vi "Main Page.vi"(8 "error in (no error)":errorcluster, 11 "Node Ptr":T1 format="%.0x") -> (0 "error out":errorcluster)   [LabVIEW 2013, in "Engine Simulation Toolkit System Explorer.lvlib"]
uses:
  Engine Simulation Toolkit System Explorer.lvlib
  <vilib>/NI Veristand/Custom Device API/Custom Device Item Ref.ctl
  <vilib>/NI Veristand/Custom Device API/Dependent File Optional Info.ctl
  System.Windows.Forms
  Shared/Properties.vi
  <vilib>/NI Veristand/Custom Device API/Get Item Property (Boolean).vi
  <vilib>/NI Veristand/Custom Device API/Get Item Property (String).vi
  <vilib>/NI Veristand/Custom Device API/Get Item Property (I32).vi
  <vilib>/NI Veristand/Custom Device API/Get Item Property (Dependent File).vi
  Shared/Constants and GUIDs.vi
  <vilib>/NI Veristand/Custom Device API/Set Item Property (String).vi
  <vilib>/NI Veristand/Custom Device API/Set Item Property (I32).vi
  <vilib>/NI Veristand/Custom Device API/Set Item Property (Dependent File).vi
  <vilib>/NI Veristand/Custom Device API/Custom Device API.lvlib
  Shared/Engine Simulation Toolkit Shared.lvlib
  <vilib>/NI Veristand/Custom Device Tools/Custom Device Utility Library/Custom Device Utility Library.lvlib
panel:
  in  "remove":bool
  in  "add":bool
  in  "APU listbox":i32[](listbox) caption="Available APUs"
  in  "Header 2":cluster{"Section Name":string}={"Section Name"="Available APUs"}
  in  "CPU":i32=-2
  out "Bitfile EPS Ver":string caption="Version of EST in bitfile"
  in  "Bitfile path":path
  in  "Device address":string="RIO0"
  in  "Rate decimation":i32=1 min=1
  in  "Execution priority":enum16{"Low", "Medium", "High"}(ring)=enum."Medium"
  out "CD Version":string caption="Custom device version"
  in  "Header":cluster{"Section Name":string}={"Section Name"="Engine Simulation Toolkit Settings"}
  in  "Name":string
  # "(-2: automatic)"
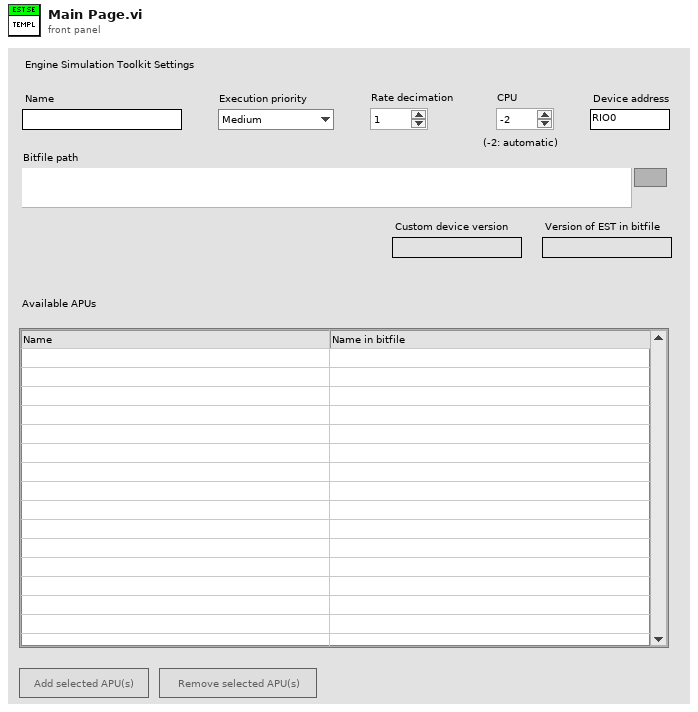
[diagram p1: front panel]
types:
  T1 = typedef "Custom Device API.lvlib/Custom Device Item Ref.ctl" = u64
  T2 = typedef "Custom Device API.lvlib/Custom Device Timed Loop Priority.ctl" = enum32{"Low", "Medium", "High"}
  T3 = typedef "Custom Device API.lvlib/Custom Device Item Info.ctl" = cluster{"Name":string, "Is Channel":bool, "GUID":string, "Is Waveform":bool}
  T4 = typedef "Custom Device API.lvlib/Dependent File Optional Info.ctl" = cluster{"Version":string, "RTDestination":path, "ForceDownload":bool, "SupportedTarget":string, "MD5":string}
  T5 = typedef "Custom Device API.lvlib/Custom Device Commands.ctl" = enum16{"Default", "Item renamed", "Shutdown", "Dynamic button pressed"}
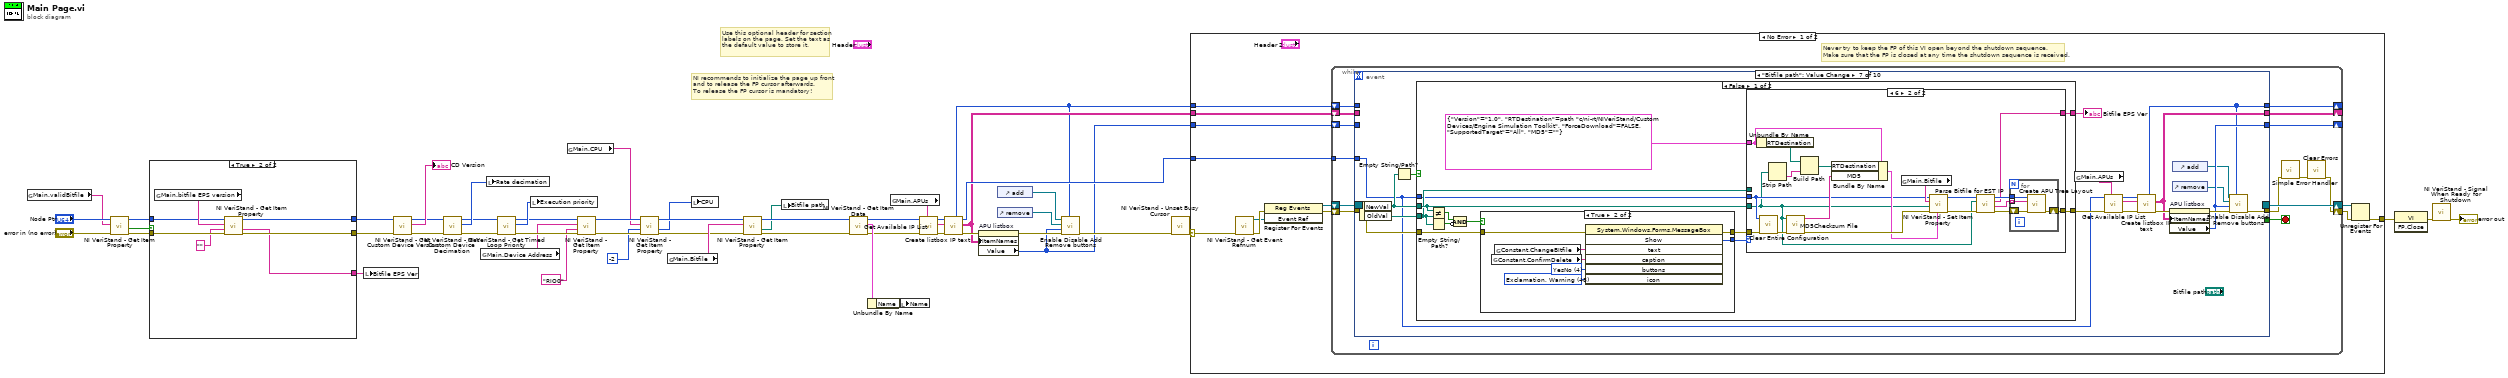
[diagram p0: block diagram]
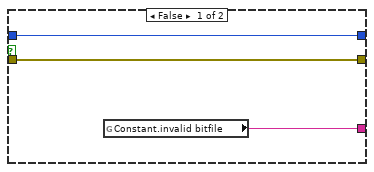
[diagram p2: hidden frame]
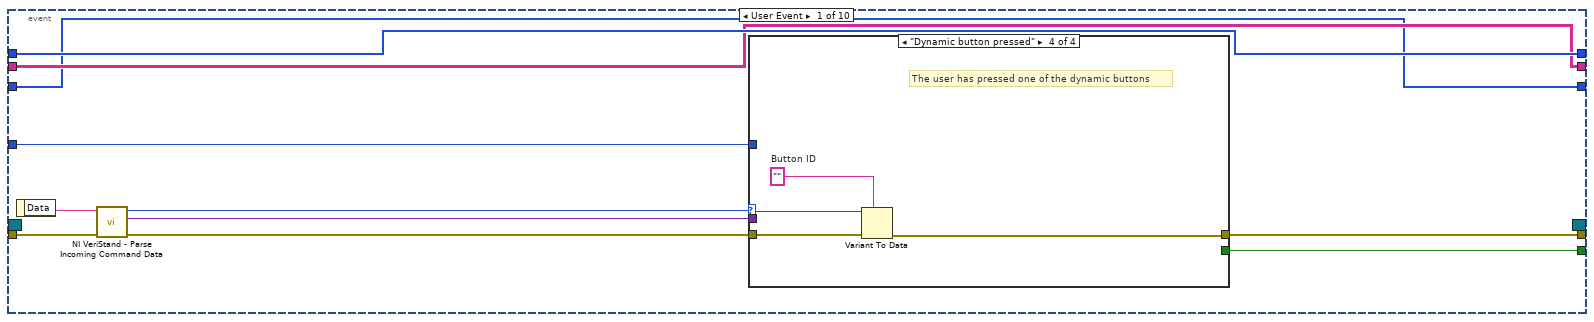
[diagram p3: hidden frame]
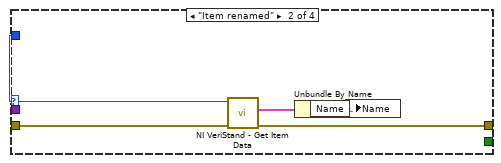
[diagram p5: hidden frame]
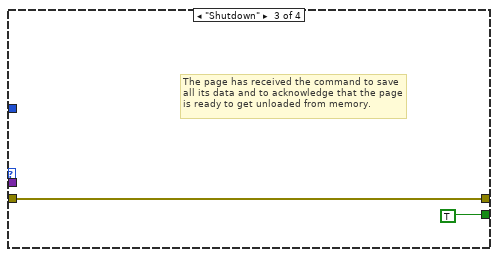
[diagram p6: hidden frame]
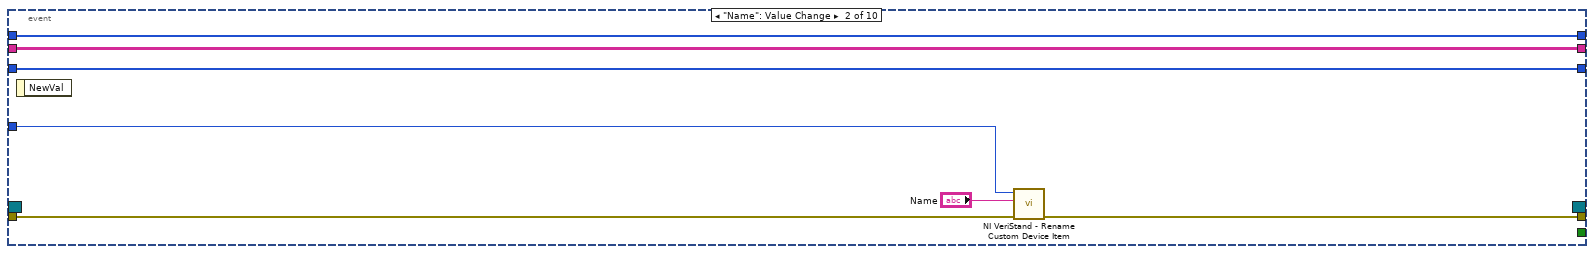
[diagram p7: hidden frame]
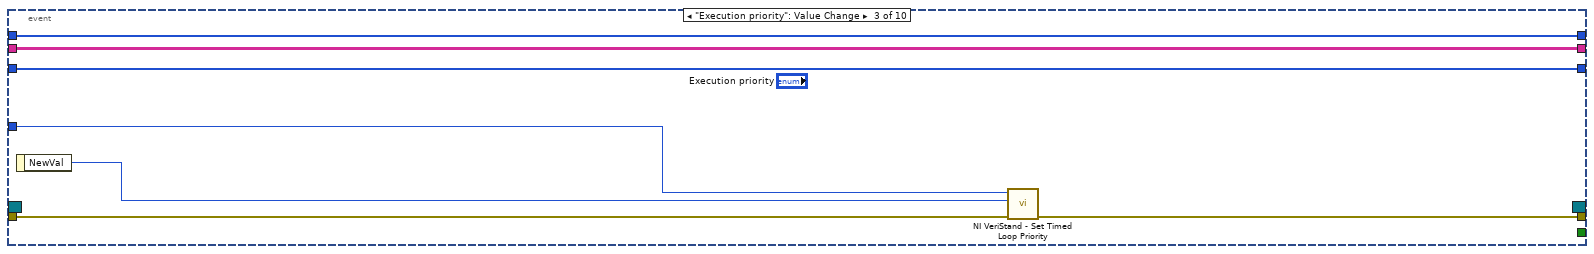
[diagram p8: hidden frame]
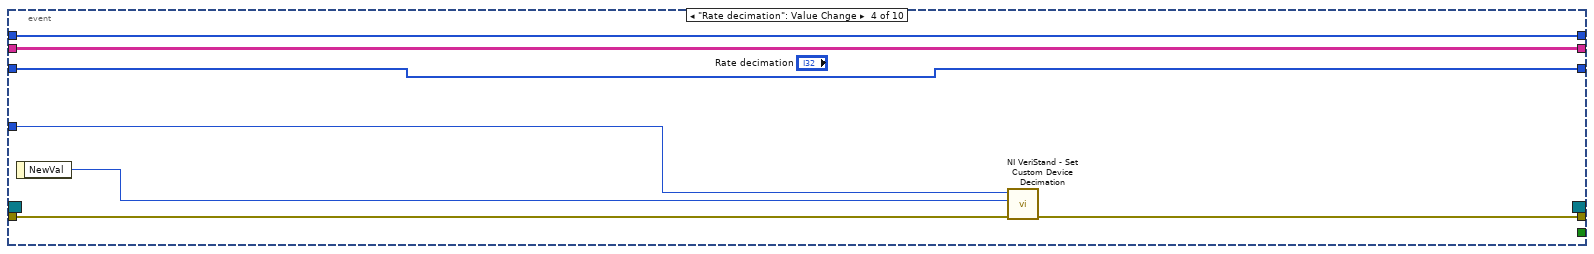
[diagram p9: hidden frame]
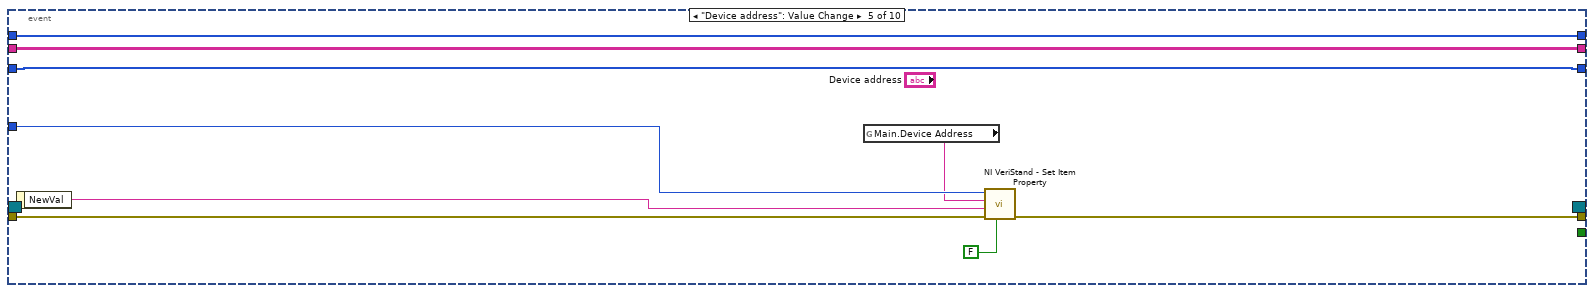
[diagram p10: hidden frame]
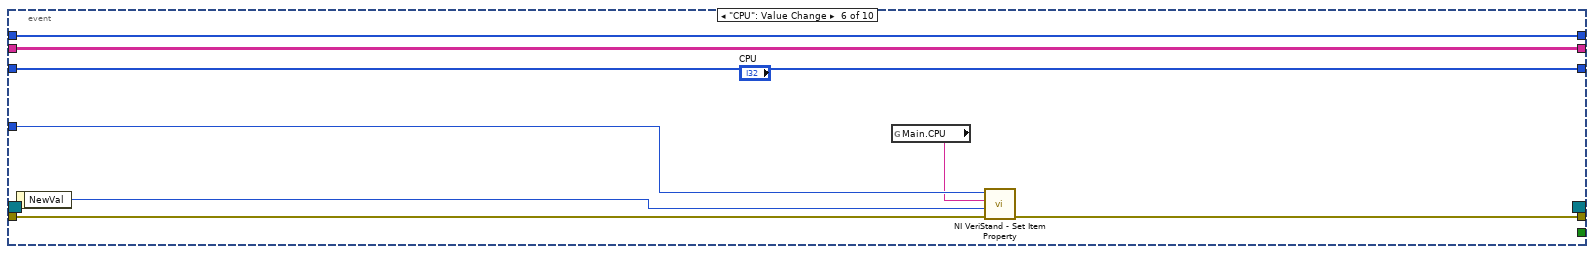
[diagram p11: hidden frame]
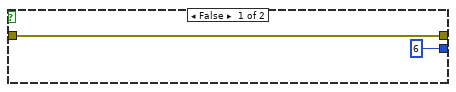
[diagram p12: hidden frame]
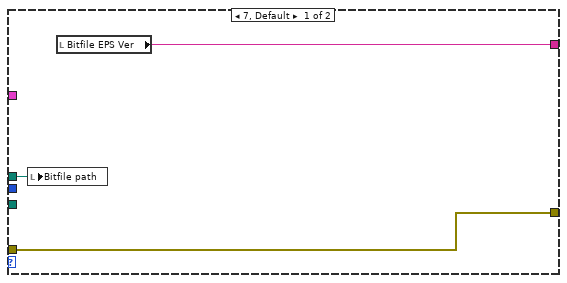
[diagram p13: hidden frame]
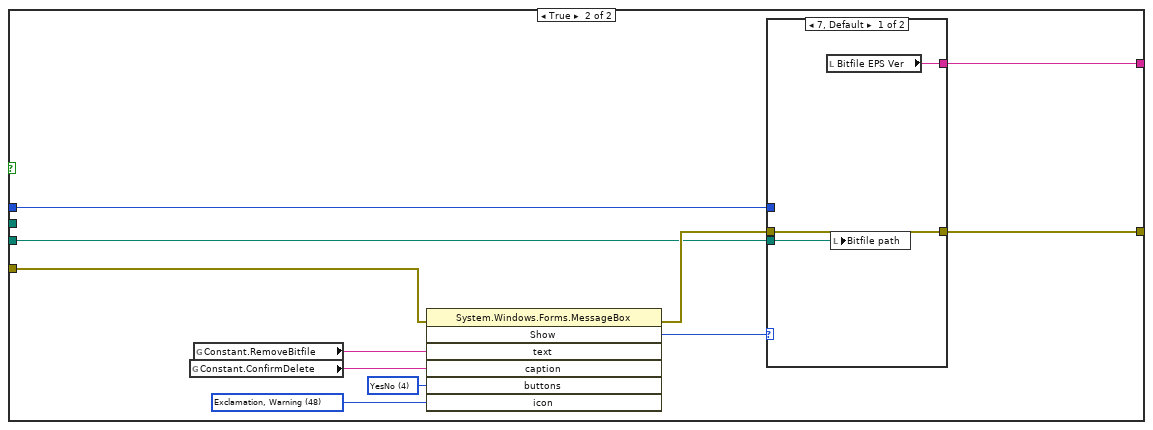
[diagram p14: hidden frame]
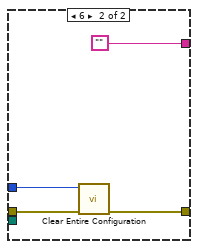
[diagram p15: hidden frame]
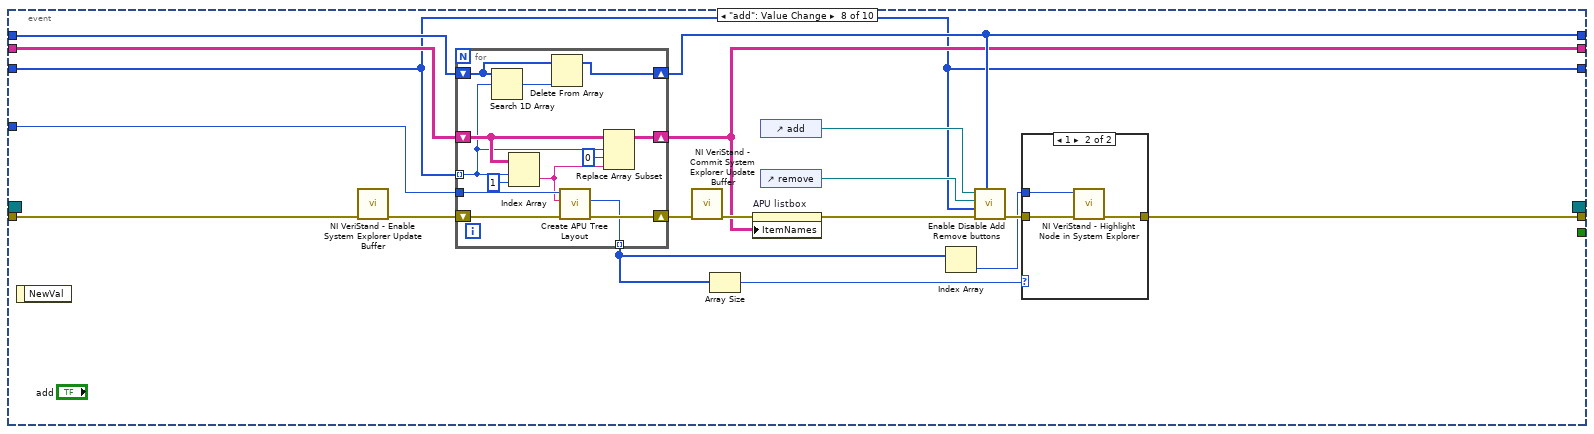
[diagram p16: hidden frame]
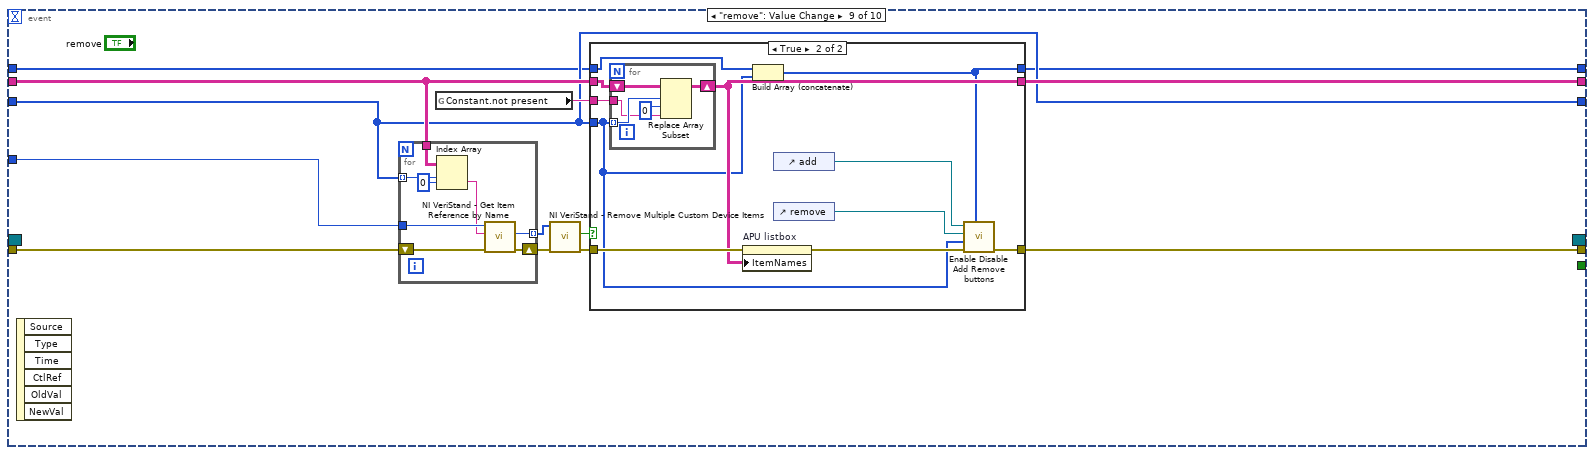
[diagram p18: hidden frame]
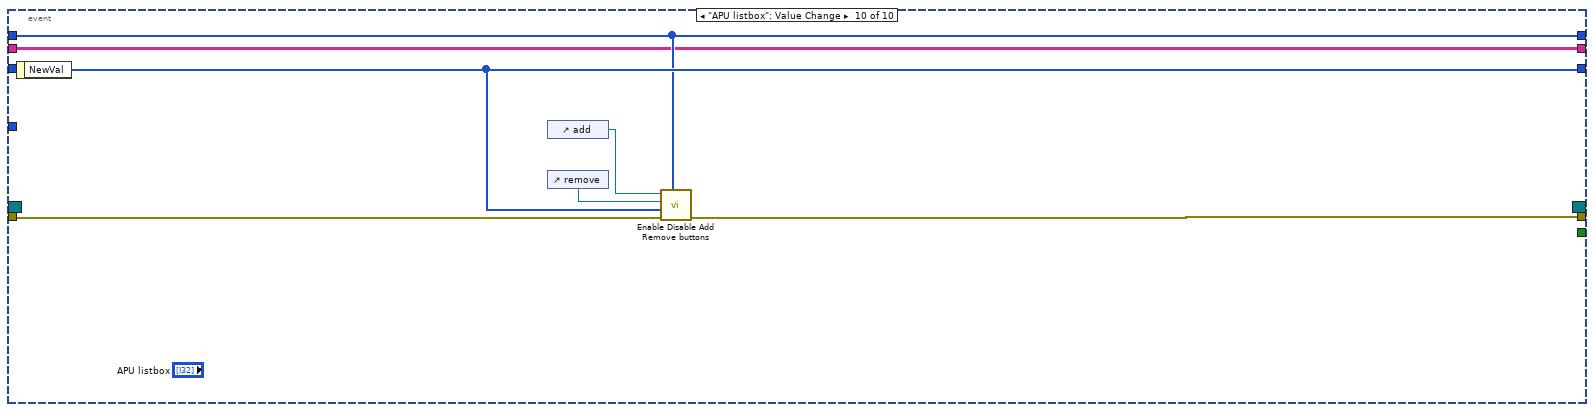
[diagram p20: hidden frame]
diagram:
  # "Use this optional header for section labels on the page. Set the text as the default value to store it."
  # "NI recommends to initialize the page up front\nand to release the FP cursor afterwards.\nTo release the FP cursor is mandatory!"
  n1 = global read "Properties.vi" "Main.validBitfile"() -> (w23:string)
  n2 = call-poly <vilib>:"NI VeriStand - Get Item Property.vi"("error in (no error)"="error in (no error)", "Property Name"=w23, "Item Ref in"="Node Ptr") -> ("error out"=w26:errorcluster, "Value"=w22:bool, "Item Ref out"=w24:T1)  [unwired: 5 in, 1 out]
  n3 = case shown="True" w22 {
    tunnel: [w55 w61] -> w29
    tunnel: [w54 w62] -> w28
    tunnel: [w53 w56] -> w27
    tunnel: w26 -> [w54 w59]
    tunnel: w24 -> [w55 w58]
    frame False {
      n4 = global read "Constants and GUIDs.vi" "Constant.invalid bitfile"() -> (w53:string)
    }
    frame True {
      n5 = global read "Properties.vi" "Main.bitfile EPS version"() -> (w60:string)
      n6 = call-poly <vilib>:"NI VeriStand - Get Item Property.vi"("error in (no error)"=w59, "Default Value"="", "Property Name"=w60, "Item Ref in"=w58) -> ("error out"=w62:errorcluster, "Value"=w56:string, "Item Ref out"=w61:T1)  [unwired: 4 in, 1 out]
    }
  }
  n7 = local write "Bitfile EPS Ver"(w27) -> ()
  n8 = call <vilib>:"NI VeriStand - Get Custom Device Version.vi"("error in (no error)"=w28, "Device Ref in"=w29) -> ("error out"=w45:errorcluster, "Value"=→"CD Version":string, "Device Ref out"=w42:T1)  [unwired: 7 in]
  n9 = call <vilib>:"NI VeriStand - Get Custom Device Decimation.vi"("error in (no error)"=w45, "Device Ref in"=w42) -> ("error out"=w43:errorcluster, "Decimation"=w41:i32, "Device Ref out"=w39:T1)  [unwired: 7 in]
  n10 = global read "Properties.vi" "Main.Device Address"() -> (w35:string)
  n11 = local write "Rate decimation"(w41) -> ()
  n12 = call <vilib>:"NI VeriStand - Get Timed Loop Priority.vi"("error in (no error)"=w43, "Device Ref in"=w39) -> ("error out"=w40:errorcluster, "Priority"=w38:T2, "Device Ref out"=w36:T1)  [unwired: 7 in]
  n13 = local write "Execution priority"(w38) -> ()
  n14 = global read "Properties.vi" "Main.CPU"() -> (w18:string)
  n15 = call-poly <vilib>:"NI VeriStand - Get Item Property.vi"("error in (no error)"=w40, "Default Value"="RIO0", "Property Name"=w35, "Item Ref in"=w36) -> ("error out"=w37:errorcluster, "Item Ref out"=w20:T1)  [unwired: 4 in, 2 out]
  n16 = call-poly <vilib>:"NI VeriStand - Get Item Property.vi"("error in (no error)"=w37, "Default Value"=-2, "Property Name"=w18, "Item Ref in"=w20) -> ("error out"=w21:errorcluster, "Value"=w16:i32, "Item Ref out"=w19:T1)  [unwired: 4 in, 1 out]
  n17 = global read "Properties.vi" "Main.Bitfile"() -> (w31:string)
  n18 = local write "CPU"(w16) -> ()
  n19 = call-poly <vilib>:"NI VeriStand - Get Item Property.vi"("error in (no error)"=w21, "Property Name"=w31, "Item Ref in"=w19) -> ("error out"=w33:errorcluster, "Path"=w30:path, "Item Ref out"=w32:T1)  [unwired: 4 in, 2 out]
  n20 = local write "Bitfile path"(w30) -> ()
  n21 = call <vilib>:"NI VeriStand - Get Item Data.vi"("error in (no error)"=w33, "Item Ref in"=w32) -> ("error out"=w6:errorcluster, "Item Info"=w47:T3, "Item Ref out"=w7:T1)  [unwired: 7 out]
  n22 = Unbundle By Name(w47) -> ("Name"=w46:string)
  n23 = global read "Properties.vi" "Main.APUs"() -> (w14:string)
  n24 = local write "Name"(w46) -> ()
  n25 = call "Get Available IP List.vi"("ip list property name"=w14, "error in (no error)"=w6, "Item Ref in"=w7) -> ("error out"=w15:errorcluster, "ips available"=w12:string[], "Item Ref out"=w13:T1)  [unwired: 6 in]
  n26 = call "Create listbox IP text.vi"("error in (no error)"=w15, "ips available"=w12, "Section Ref in"=w13) -> ("error out"=w11:errorcluster, "listbox text"=w3:string[][], "Section Ref out"=w4:T1, "not present item indexes"=w2:i32[])  [unwired: 5 in]
  n27 = property on="APU listbox" class="MCListbox (strict)"(error in=w11, "ItemNames"=w3) -> (error out=w8:errorcluster, "Value"=w1:i32[])  [unwired: 1 in, 1 out]
  n28 = control-ref of="add"() -> (w9:refnum<vi>)
  n29 = control-ref of="remove"() -> (w10:refnum<vi>)
  n30 = call "Enable Disable Add Remove buttons.vi"("not present item indexes"=w2, "error in (no error)"=w8, "selected items"=w1, "remove button"=w10, "add button"=w9) -> ("error out"=w5:errorcluster)  [unwired: 6 in]
  n31 = call <vilib>:"NI VeriStand - Unset Busy Cursor.vi"("error in (no error)"=w5) -> ("error out"=w49:errorcluster)  [unwired: 10 out]
  n32 = case shown="No Error" w49 {
    selector: w49 -> [w66 w318]
    tunnel: [w71 w316] -> w52
    tunnel: w4 -> [w67 _]
    tunnel: w3 -> [w65 _]
    tunnel: w2 -> [w64 _]
    tunnel: w1 -> [w63 _]
    frame No Error {
      # "Never try to keep the FP of this VI open beyond the shutdown sequence.\nMake sure that the FP is closed at any time the shutdown sequence is received."
      n33 = call <vilib>:"NI VeriStand - Get Event Refnum.vi"("error in (no error)"=w66) -> ("error out"=w74:errorcluster, "Event Ref"=w70:refnum<user-event>)  [unwired: 9 out]
      n34 = register-events(error in=w74, w70) -> (reference out=w68:refnum<event-registration>, error out=w69:errorcluster)  [unwired: 1 in]
      n35 = while {
        tunnel: w67 -> [w84]
        shift-right: [w81] -> w72
        shift-left: w69 -> [w87]
        shift-right: [w88] -> w73
        shift-left: w68 -> [w86]
        shift-right: [w75] -> _
        shift-left: w63 -> [w78]
        shift-right: [w76] -> _
        shift-left: w65 -> [w80]
        shift-right: [w77] -> _
        shift-left: w64 -> [w79]
        stop <- w85 stop-if-true
        n36 = event shown="[6] \"Bitfile path\": Value Change" {
          selector: w86 -> [_ _ _ _ _ _ _ _ _ _]
          dyn-events: [_ _ _ _ _ _ _ _ _ _] -> w88
          timeout: _ -> [_ _ _ _ _ _ _ _ _ _]
          tunnel: w87 -> [w99 w118 w125 w132 w141 w149 w168 w241 w276 w313]
          tunnel: [w95 _ _ _ _ _ _ _ _ _] -> w85
          tunnel: [w94 w117 w123 w130 w137 w145 w160 w240 w275 w312] -> w83
          tunnel: w84 -> [w93 w116 w124 w131 w140 w148 w152 w237 w271 _]
          tunnel: w80 -> [w90 w113 w120 w127 w134 w143 _ w238 w274 w309]
          tunnel: w79 -> [w91 w114 w121 w128 w135 w144 _ w239 w270 w310]
          tunnel: w78 -> [w89 w112 w119 w126 w133 w142 _ w234 w272 _]
          tunnel: [w91 w114 w121 w128 w135 w144 w158 w236 w269 w310] -> w77
          tunnel: [w90 w113 w120 w127 w134 w143 w162 w235 w273 w309] -> w76
          tunnel: [w89 w112 w119 w126 w133 w142 w159 w234 w272 w311] -> w75
          event User Event {
            n37 = event-data() -> ("Data"=w98:string)  [unwired: 1 out]
            n38 = call <vilib>:"NI VeriStand - Parse Incoming Command Data.vi"("error in (no error)"=w99, "Incoming data"=w98) -> ("error out"=w97:errorcluster, "Outgoing data"=w92:variant, "Action"=w96:T5)  [unwired: 7 out]
            n39 = case shown="\"Dynamic button pressed\"" w96 {
              tunnel: w97 -> [w100 w105 w106 w111]
              tunnel: [_ _ TRUE _] -> w95
              tunnel: [w100 w102 w106 w108] -> w94
              tunnel: w93 -> [_ w104 _ _]
              tunnel: w92 -> [_ _ _ w110]
              frame "Default", Default {
              }
              frame "Item renamed" {
                n40 = call <vilib>:"NI VeriStand - Get Item Data.vi"("error in (no error)"=w105, "Item Ref in"=w104) -> ("error out"=w102:errorcluster, "Item Info"=w103:T3)  [unwired: 8 out]
                n41 = Unbundle By Name(w103) -> ("Name"=w101:string)
                n42 = local write "Name"(w101) -> ()
              }
              frame "Shutdown" {
                # "The page has received the command to save all its data and to acknowledge that the page is ready to get unloaded from memory."
              }
              frame "Dynamic button pressed" {
                w109 = ""  # Button ID
                # "The user has pressed one of the dynamic buttons"
                n43 = Variant To Data(error in=w111, type=w109, Variant=w110) -> (error out=w108:errorcluster)  [unwired: 1 out]
              }
            }
          }
          event "Name": Value Change {
            n44 = event-data() -> ()  [unwired: 2 out]
            n45 = call <vilib>:"NI VeriStand - Rename Custom Device Item.vi"("error in (no error)"=w118, "New Name"="Name", "Item Ref in"=w116) -> ("error out"=w117:errorcluster)  [unwired: 1 in, 7 out]
          }
          event "Execution priority": Value Change {
            n46 = event-data() -> ("NewVal"=w122:enum16{"Low", "Medium", "High"})  [unwired: 1 out]
            n47 = call <vilib>:"NI VeriStand - Set Timed Loop Priority.vi"("error in (no error)"=w125, "Priority"=w122, "Device Ref in"=w124) -> ("error out"=w123:errorcluster)  [unwired: 7 in, 1 out]
          }
          event "Rate decimation": Value Change {
            n48 = event-data() -> ("NewVal"=w129:i32)  [unwired: 1 out]
            n49 = call <vilib>:"NI VeriStand - Set Custom Device Decimation.vi"("error in (no error)"=w132, "Decimation"=w129, "Device Ref in"=w131) -> ("error out"=w130:errorcluster)  [unwired: 7 in, 1 out]
          }
          event "Device address": Value Change {
            n50 = event-data() -> ("NewVal"=w139:string)  [unwired: 1 out]
            n51 = global read "Properties.vi" "Main.Device Address"() -> (w138:string)
            n52 = call-poly <vilib>:"NI VeriStand - Set Item Property.vi"("Binary String (T)"=FALSE, "error in (no error)"=w141, "Value"=w139, "Property Name"=w138, "Item Ref in"=w140) -> ("error out"=w137:errorcluster)  [unwired: 4 in, 2 out]
          }
          event "CPU": Value Change {
            n53 = event-data() -> ("NewVal"=w147:i32)  [unwired: 1 out]
            n54 = global read "Properties.vi" "Main.CPU"() -> (w146:string)
            n55 = call-poly <vilib>:"NI VeriStand - Set Item Property.vi"("error in (no error)"=w149, "Value"=w147, "Property Name"=w146, "Item Ref in"=w148) -> ("error out"=w145:errorcluster)  [unwired: 5 in, 2 out]
          }
          event "Bitfile path": Value Change {
            n56 = event-data() -> ("NewVal"=w165:path, "OldVal"=w164:path)  [unwired: 1 out]
            n57 = Empty String/Path?(string/path=w165) -> (empty?=w166:bool)
            n58 = case shown="False" w166 {
              tunnel: w152 -> [w170 w226]
              tunnel: w168 -> [w174 w222]
              tunnel: w165 -> [w178 _]
              tunnel: [w179 w225] -> w154
              tunnel: [w180 w219] -> w167
              tunnel: w164 -> [w171 w218]
              frame False {
                n59 = Not Equal?(x=w178, y=w171) -> (x != y?=w177:bool)
                n60 = Empty String/Path?(string/path=w171) -> (empty?=w176:bool)
                n61 = Compound Arithmetic op=AND(w177, invert w176) -> (w175:bool)
                n62 = case shown="True" w175 {
                  tunnel: w174 -> [w182 w185]
                  tunnel: [6 ("Show") w184] -> w173
                  tunnel: [w182 w183] -> w172
                  frame False {
                  }
                  frame True {
                    w189 = 4 items=["OK", "OKCancel", "AbortRetryIgnore", "YesNoCancel", "YesNo", "RetryCancel"] ("buttons")
                    w188 = 48 items=["None"=0, "Hand, Error, Stop"=16, "Question"=32, "Exclamation, Warning"=48, "Asterisk, Information"=64] ("icon")
                    n63 = global read "Constants and GUIDs.vi" "Constant.ConfirmDelete"() -> (w186:string)
                    n64 = global read "Constants and GUIDs.vi" "Constant.ChangeBItfile"() -> (w187:string)
                    n65 = invoke class="System.Windows.Forms.MessageBox" method="Show"(error in=w185, "text"=w187, "caption"=w186, "buttons"=w189, "icon"=w188) -> (error out=w183:errorcluster, "Show"=w184:i32)  [unwired: 2 in, 5 out]
                  }
                }
                n66 = case shown="6" w173 {
                  tunnel: w170 -> [_ w200]
                  tunnel: w172 -> [w192 w202]
                  tunnel: [w190 w198] -> w180
                  tunnel: [w192 w206] -> w179
                  tunnel: w178 -> [_ w196]
                  tunnel: w171 -> [w191 _]
                  tunnel: T4 {"Version"="1.0", "RTDestination"=path "c:/ni-rt/NIVeriStand/Custom Devices/Engine Simulation Toolkit", "ForceDownload"=FALSE, "SupportedTarget"="All", "MD5"=""} ("OptionalInfo") -> [_ w197]
                  frame 7, Default {
                    n67 = local write "Bitfile path"(w191) -> ()
                    n68 = local read "Bitfile EPS Ver"() -> (w190:string)
                  }
                  frame 6 {
                    n69 = Unbundle By Name(w197) -> ("RTDestination"=w195:path)
                    n70 = call "Clear Entire Configuration.vi"("error in (no error)"=w202, "Item Ref in"=w200) -> ("error out"=w201:errorcluster)  [unwired: 9 in]
                    n71 = Strip Path(path=w196) -> (name=w193:string)  [unwired: 1 out]
                    n72 = call <vilib>:"MD5Checksum File.vi"("error in (no error)"=w201, "Path"=w196) -> ("error out"=w210:errorcluster, "MD5 message-digest"=w209:string)  [unwired: 8 in]
                    n73 = Build Path(base path=w195, name or relative path=w193) -> (appended path=w194:path)
                    n74 = Bundle By Name(cluster=w197, "RTDestination"=w194, "MD5"=w209) -> (w208:T4)
                    n75 = global read "Properties.vi" "Main.Bitfile"() -> (w203:string)
                    n76 = call-poly <vilib>:"NI VeriStand - Set Item Property.vi"("OptionalInfo"=w208, "error in (no error)"=w210, "Path"=w196, "Property Name"=w203, "Item Ref in"=w200) -> ("error out"=w211:errorcluster, "Item Ref out"=w207:T1)  [unwired: 4 in, 1 out]
                    n77 = call "Parse Bitfile for EST IP.vi"("error in (no error)"=w211, "bitfile path"=w196, "Item Ref in"=w207) -> ("error out"=w199:errorcluster, "APUs"=w204:string[], "version"=w198:string, "Item Ref out"=w205:T1)  [unwired: 5 in]
                    n78 = for {
                      shift-right: [w214] -> w206
                      shift-left: w199 -> [w215]
                      tunnel: w205 -> [w213]
                      tunnel: w204 -> [w212] mode=indexing
                      n79 = call "Create APU Tree Layout.vi"("error in (no error)"=w215, "engine name"=w212, "Section Ptr"=w213) -> ("error out"=w214:errorcluster)  [unwired: 6 in, 2 out]
                    }
                  }
                }
              }
              frame True {
                w224 = 4 items=["OK", "OKCancel", "AbortRetryIgnore", "YesNoCancel", "YesNo", "RetryCancel"] ("buttons")
                w223 = 48 items=["None"=0, "Hand, Error, Stop"=16, "Question"=32, "Exclamation, Warning"=48, "Asterisk, Information"=64] ("icon")
                n80 = global read "Constants and GUIDs.vi" "Constant.ConfirmDelete"() -> (w216:string)
                n81 = global read "Constants and GUIDs.vi" "Constant.RemoveBitfile"() -> (w217:string)
                n82 = invoke class="System.Windows.Forms.MessageBox" method="Show"(error in=w222, "text"=w217, "caption"=w216, "buttons"=w224, "icon"=w223) -> (error out=w221:errorcluster, "Show"=w220:i32)  [unwired: 2 in, 5 out]
                n83 = case shown="7, Default" w220 {
                  tunnel: w226 -> [_ w233]
                  tunnel: [w229 w230] -> w225
                  tunnel: w221 -> [w229 w232]
                  tunnel: [w228 ""] -> w219
                  tunnel: w218 -> [w227 _]
                  frame 7, Default {
                    n84 = local read "Bitfile EPS Ver"() -> (w228:string)
                    n85 = local write "Bitfile path"(w227) -> ()
                  }
                  frame 6 {
                    n86 = call "Clear Entire Configuration.vi"("error in (no error)"=w232, "Item Ref in"=w233) -> ("error out"=w230:errorcluster)  [unwired: 9 in]
                  }
                }
              }
            }
            "Bitfile EPS Ver" <- w167
            n87 = global read "Properties.vi" "Main.APUs"() -> (w155:string)
            n88 = call "Get Available IP List.vi"("ip list property name"=w155, "error in (no error)"=w154, "Item Ref in"=w152) -> ("error out"=w153:errorcluster, "ips available"=w150:string[], "Item Ref out"=w151:T1)  [unwired: 6 in]
            n89 = call "Create listbox IP text.vi"("error in (no error)"=w153, "ips available"=w150, "Section Ref in"=w151) -> ("error out"=w163:errorcluster, "listbox text"=w162:string[][], "not present item indexes"=w158:i32[])  [unwired: 5 in, 1 out]
            n90 = property on="APU listbox" class="MCListbox (strict)"(error in=w163, "ItemNames"=w162) -> (error out=w161:errorcluster, "Value"=w159:i32[])  [unwired: 1 in, 1 out]
            n91 = control-ref of="add"() -> (w156:refnum<vi>)
            n92 = control-ref of="remove"() -> (w157:refnum<vi>)
            n93 = call "Enable Disable Add Remove buttons.vi"("not present item indexes"=w158, "error in (no error)"=w161, "selected items"=w159, "remove button"=w157, "add button"=w156) -> ("error out"=w160:errorcluster)  [unwired: 6 in]
          }
          event "add": Value Change {
            n94 = event-data() -> ()  [unwired: 2 out]
            n95 = call <vilib>:"NI VeriStand - Enable System Explorer Update Buffer.vi"("error in (no error)"=w241) -> ("error out"=w246:errorcluster)  [unwired: 10 in]
            n96 = for {
              tunnel: w237 -> [w266]
              shift-right: [w267] -> w251
              shift-left: w246 -> [w268]
              tunnel: w234 -> [w260] mode=indexing
              shift-right: [w263] -> w235
              shift-left: w238 -> [w264]
              shift-right: [w257] -> w236
              shift-left: w239 -> [w259]
              tunnel: [w256] -> w244 mode=indexing
              n97 = Search 1D Array(1D array=w259, element=w260) -> (index of element=w258:i32)  [unwired: 1 in]
              n98 = Index Array(array=w264, index (row)=w260, index (col)=1 ("disabled index (col)")) -> (element=w261:string)
              n99 = Delete From Array(array=w259, index=w258) -> (array with subset deleted=w257:i32[])  [unwired: 1 in, 1 out]
              n100 = call "Create APU Tree Layout.vi"("error in (no error)"=w268, "engine name"=w261, "Section Ptr"=w266) -> ("error out"=w267:errorcluster, "APU ref"=w256:T1)  [unwired: 6 in, 1 out]
              n101 = Replace Array Subset(array=w264, new element=w261, index (row)=w260, index (col)=0 ("disabled index (col)")) -> (w263:string[][])
            }
            n102 = call <vilib>:"NI VeriStand - Commit System Explorer Update Buffer.vi"("error in (no error)"=w251) -> ("error out"=w245:errorcluster)  [unwired: 10 in]
            n103 = Array Size(array=w244) -> (size(s)=w242:i32)
            n104 = property on="APU listbox" class="MCListbox (strict)"(error in=w245, "ItemNames"=w235) -> (error out=w250:errorcluster)  [unwired: 1 in, 1 out]
            n105 = control-ref of="add"() -> (w248:refnum<vi>)
            n106 = control-ref of="remove"() -> (w247:refnum<vi>)
            n107 = Index Array(array=w244) -> (element=w243:T1)  [unwired: 1 in]
            n108 = call "Enable Disable Add Remove buttons.vi"("not present item indexes"=w236, "error in (no error)"=w250, "selected items"=w234, "remove button"=w247, "add button"=w248) -> ("error out"=w249:errorcluster)  [unwired: 6 in]
            n109 = case shown="1" w242 {
              tunnel: w249 -> [w252 w253]
              tunnel: [w252 w255] -> w240
              tunnel: w243 -> [_ w254]
              frame Default {
              }
              frame 1 {
                n110 = call <vilib>:"NI VeriStand - Highlight Node in System Explorer.vi"("error in (no error)"=w253, "Item Ref in"=w254) -> ("error out"=w255:errorcluster)  [unwired: 8 in, 1 out]
              }
            }
          }
          event "remove": Value Change {
            n111 = event-data() -> ()  [unwired: 7 out]
            n112 = for {
              tunnel: w272 -> [w307] mode=indexing
              tunnel: w274 -> [w308]
              tunnel: w271 -> [w304]
              tunnel: [w301] -> w280 mode=indexing
              shift-right: [w303] -> w281
              shift-left: w276 -> [w305]
              n113 = Index Array(array=w308, index (row)=w307, index (col)=0 ("disabled index (col)")) -> (element=w302:string)
              n114 = call <vilib>:"NI VeriStand - Get Item Reference by Name.vi"("error in (no error)"=w305, "Item Name"=w302, "Parent Ref in"=w304) -> ("error out"=w303:errorcluster, "Item Ref"=w301:T1)  [unwired: 5 in, 2 out]
            }
            n115 = global read "Constants and GUIDs.vi" "Constant.not present"() -> (w277:string)
            n116 = call <vilib>:"NI VeriStand - Remove Multiple Custom Device Items.vi"("error in (no error)"=w281, "Item Refs in"=w280) -> ("error out"=w279:errorcluster, "Deleted?"=w278:bool)  [unwired: 8 in]
            n117 = case shown="True" w278 {
              tunnel: [w283 w294] -> w275
              tunnel: w279 -> [w283 w291]
              tunnel: w272 -> [_ w286]
              tunnel: w274 -> [w284 w290]
              tunnel: w277 -> [_ w289]
              tunnel: [w284 w288] -> w273
              tunnel: w270 -> [w282 w287]
              tunnel: [w282 w285] -> w269
              frame False {
              }
              frame True {
                n118 = for {
                  tunnel: w286 -> [w298] mode=indexing
                  shift-right: [w299] -> w288
                  shift-left: w290 -> [w300]
                  tunnel: w289 -> [w296]
                  n119 = Replace Array Subset(array=w300, new element=w296, index (row)=w298, index (col)=0 ("disabled index (col)")) -> (w299:string[][])
                }
                n120 = property on="APU listbox" class="MCListbox (strict)"(error in=w291, "ItemNames"=w288) -> (error out=w295:errorcluster)  [unwired: 1 in, 1 out]
                n121 = Build Array (concatenate)(w287, w286) -> (w285:i32[])
                n122 = control-ref of="add"() -> (w293:refnum<vi>)
                n123 = control-ref of="remove"() -> (w292:refnum<vi>)
                n124 = call "Enable Disable Add Remove buttons.vi"("not present item indexes"=w285, "error in (no error)"=w295, "selected items"=w286, "remove button"=w292, "add button"=w293) -> ("error out"=w294:errorcluster)  [unwired: 6 in]
              }
            }
          }
          event "APU listbox": Value Change {
            n125 = event-data() -> ("NewVal"=w311:i32[])  [unwired: 1 out]
            n126 = control-ref of="add"() -> (w315:refnum<vi>)
            n127 = control-ref of="remove"() -> (w314:refnum<vi>)
            n128 = call "Enable Disable Add Remove buttons.vi"("not present item indexes"=w310, "error in (no error)"=w313, "selected items"=w311, "remove button"=w314, "add button"=w315) -> ("error out"=w312:errorcluster)  [unwired: 6 in]
          }
        }
        n129 = call <vilib>:"Simple Error Handler.vi"("error in (no error)"=w83) -> ("error out"=w82:errorcluster)  [unwired: 1 in, 7 out]
        n130 = call <vilib>:"Clear Errors.vi"("error in (no error)"=w82) -> ("error out"=w81:errorcluster)  [unwired: 6 out]
      }
      n131 = Unregister For Events(event registration refnum=w73, error in=w72) -> (error out=w71:errorcluster)
    }
    frame Error {
      n132 = call <vilib>:"Simple Error Handler.vi"("error in (no error)"=w318) -> ("error out"=w317:errorcluster)  [unwired: 1 in, 7 out]
      n133 = call <vilib>:"Clear Errors.vi"("error in (no error)"=w317) -> ("error out"=w316:errorcluster)  [unwired: 6 out]
    }
  }
  n134 = invoke class="VI" method="FP.Close"(error in=w52) -> (error out=w51:errorcluster)  [unwired: 2 in, 2 out]
  n135 = call <vilib>:"NI VeriStand - Signal When Ready for Shutdown.vi"("error in (no error)"=w51) -> ("error out"=→"error out":errorcluster)  [unwired: 10 out]
